vi "LookupBadgeName.vi"(8 "error in (no error)":errorcluster, 11 "badgename":string="ljj1838") -> (0 "error out":errorcluster, 2 "return type":u32, 3 "fullname":string)   [LabVIEW 2019]
doc: "Get the full user name from a scanned badge name"
uses:
  LVWinFun.dll
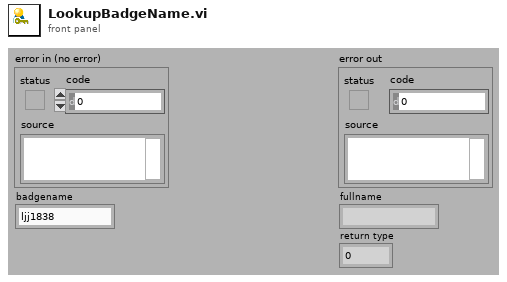
[diagram p1: front panel]
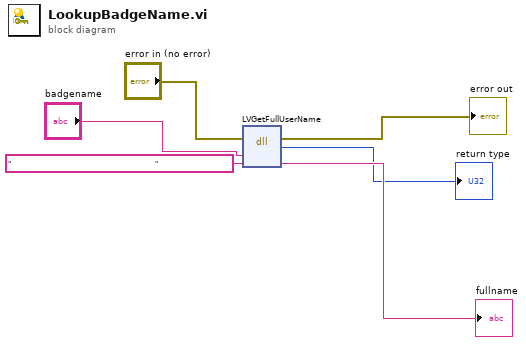
[diagram p0: block diagram]
diagram:
  n1 = dll-call lib="F:/src/HUTCDLSVN/Machine/CDL0100/HMI/Support VIs/LVWinFun.dll" fn="LVGetFullUserName"(error in="error in (no error)", "badgename"="badgename", "fullname"="                                                                        ") -> (error out=→"error out":errorcluster, "return type"=→"return type":u32, "fullname"=→"fullname":string)  [unwired: 3 in, 1 out]
